vi "Test.vi"() -> ()   [LabVIEW 2018]
uses:
  <vilib>/ethernetip/ethernetip.llb/EthernetIPSLC500FileType.ctl
  <vilib>/ethernetip/ethernetip.llb/EthernetIP SLC500 Read Raw.vi
  <vilib>/ethernetip/ethernetip.llb/EthernetIP SLC500 Write Raw.vi
  <vilib>/ethernetip/ethernetip.llb/EthernetIP SLC500 Write Bit.vi
  <vilib>/ethernetip/ethernetip.lvlib
panel:
  in  "Element Number  2":u16
  in  "Element Number":u16=1
  in  "Bits":bool[](array[boolean])
  in  "Hex Data":u8[](array[numeric]) format="%.0x"
  in  "stop":bool
  out "Input":bool[](array[boolean])
  out "error out":errorcluster
  in  "IP Address":string
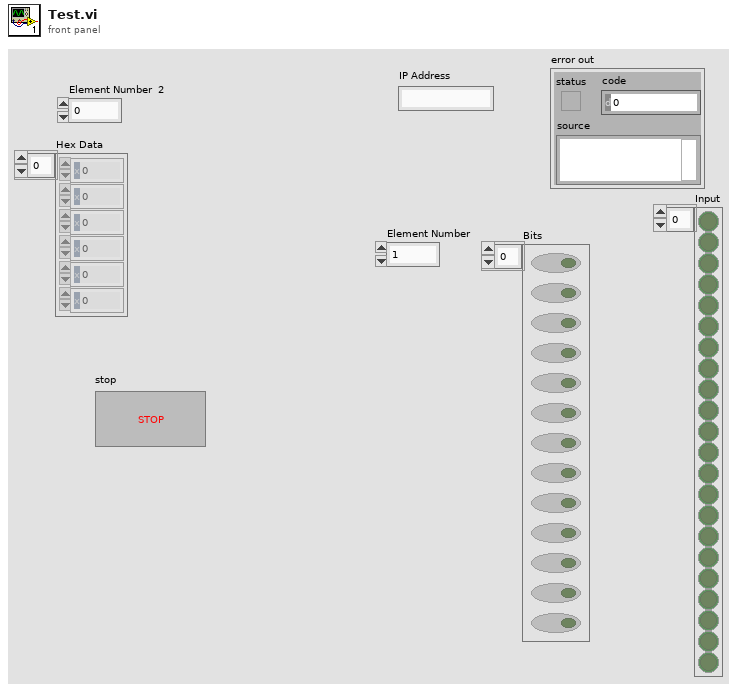
[diagram p1: front panel]
types:
  T1 = typedef "ethernetip.lvlib/ethernetip.ctl" = refnum<k21>
  T2 = typedef "ethernetip.lvlib/EthernetIPSLC500FileType.ctl" = u8
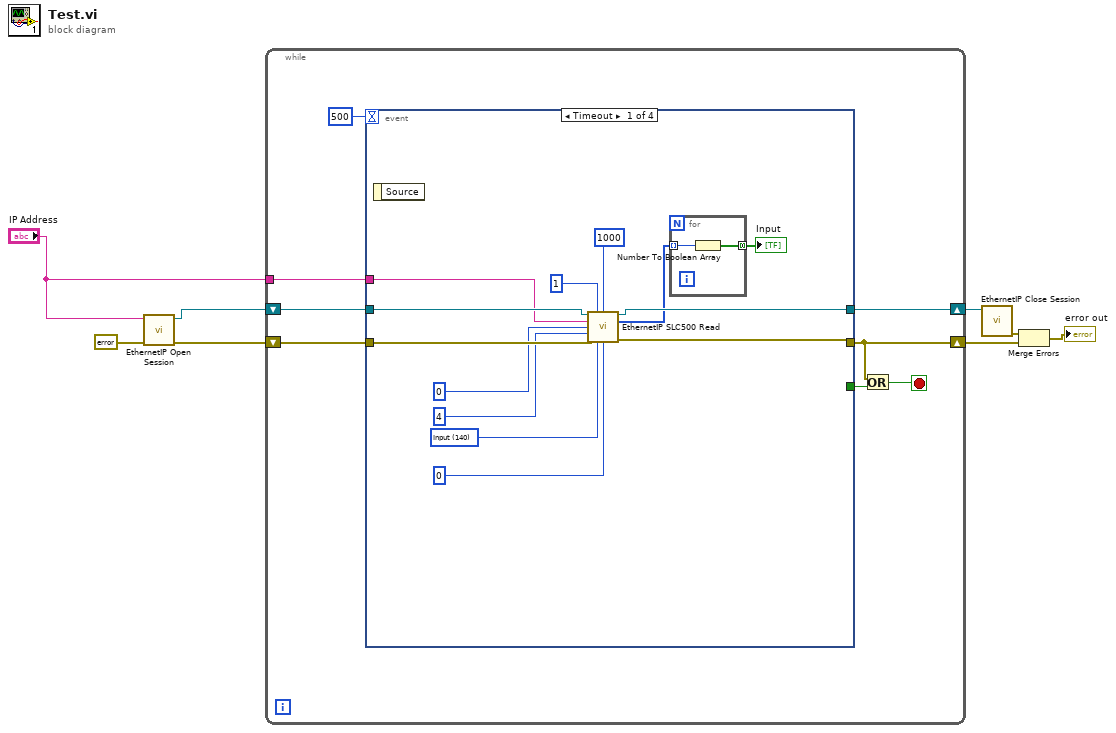
[diagram p0: block diagram]
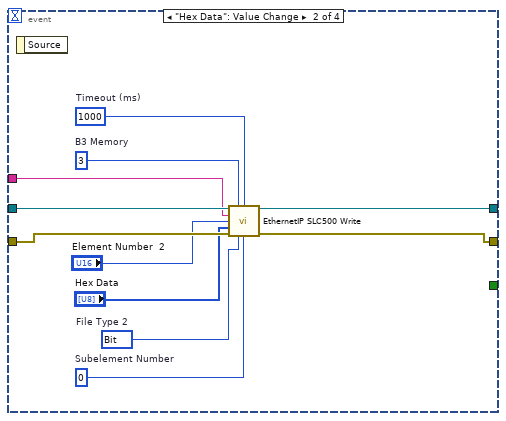
[diagram p2: hidden frame]
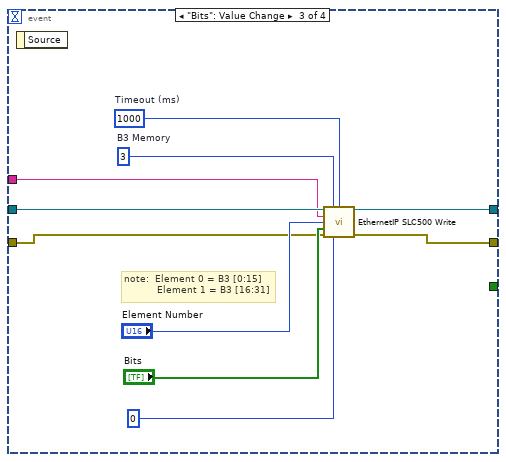
[diagram p3: hidden frame]
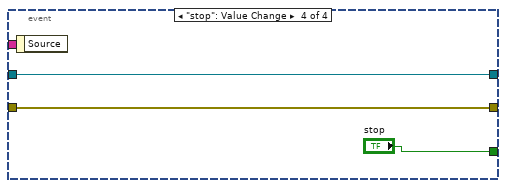
[diagram p4: hidden frame]
diagram:
  n1 = call <vilib>:"EthernetIP Open Session.vi"("error in"=errorcluster {"status"=FALSE, "code"=0, "source"=""} ("error in (no error)"), "Session in"="IP Address") -> ("error out"=w4:errorcluster, "Session out"=w3:T1)  [unwired: 8 in]
  n2 = while {
    shift-right: [w10] -> w6
    shift-left: w4 -> [w13]
    shift-right: [w11] -> w2
    shift-left: w3 -> [w12]
    tunnel: "IP Address" -> [w9]
    stop <- w14 stop-if-true
    n3 = event shown="[0] Timeout" {
      selector: _ -> [_ _ _ _]
      dyn-events: _ -> [_ _ _ _]
      timeout: 500 -> [_ _ _ _]
      tunnel: [_ _ _ "stop"] -> w15
      tunnel: w13 -> [w28 w40 w47 w54]
      tunnel: [w26 w39 w46 w54] -> w10
      tunnel: w12 -> [w29 w42 w50 w53]
      tunnel: [w27 w41 w49 w53] -> w11
      tunnel: w9 -> [w25 w36 w48 _]
      event Timeout {
        w18 = T2 140 items=["Status"=132, "Bit"=133, "Timer"=134, "Counter"=135, "Control"=136, "Integer"=137, "Float"=138, "Output"=139, "Input"=140, "String"=141, "ASCII"=142] ("File Type")
        n4 = event-data() -> ()  [unwired: 1 in, 1 out]
        n5 = call-poly <vilib>:"EthernetIP SLC500 Read.vi"("Session in"=w29, "File Number"=u16 1, "Timeout (ms)"=1000, "Network Path"=w25, "Element Number"=u16 0, "Number of Bytes"=u32 4, "error in"=w28, "File Type"=w18, "Subelement Number"=u16 0) -> ("Session out"=w27:T1, "Data"=w21:u8[], "error out"=w26:errorcluster)  [unwired: 4 in]
        n6 = for {
          tunnel: w21 -> [w31] mode=indexing
          tunnel: [w30] -> w22 mode=concatenating
          n7 = Number To Boolean Array(number=w31) -> (Boolean array=w30:bool[])
        }
        "Input" <- w22
      }
      event "Hex Data": Value Change {
        w32 = u16 0  # Subelement Number
        w33 = T2 133 items=["Status"=132, "Bit"=133, "Timer"=134, "Counter"=135, "Control"=136, "Integer"=137, "Float"=138, "Output"=139, "Input"=140, "String"=141, "ASCII"=142]  # File Type 2
        w37 = u16 3  # B3 Memory
        w38 = 1000  # Timeout (ms)
        n8 = event-data() -> ()  [unwired: 1 in, 1 out]
        n9 = call-poly <vilib>:"EthernetIP SLC500 Write.vi"("Session in"=w42, "File Number"=w37, "Timeout (ms)"=w38, "Network Path"=w36, "Element Number"="Element Number  2", "Data"="Hex Data", "error in"=w40, "File Type"=w33, "Subelement Number"=w32) -> ("Session out"=w41:T1, "error out"=w39:errorcluster)  [unwired: 5 in]
      }
      event "Bits": Value Change {
        w44 = 1000  # Timeout (ms)
        w45 = u16 3  # B3 Memory
        # "note:  Element 0 = B3 [0:15]\n           Element 1 = B3 [16:31]"
        n10 = event-data() -> ()  [unwired: 1 in, 1 out]
        n11 = call-poly <vilib>:"EthernetIP SLC500 Write.vi"("Session in"=w50, "File Number"=w45, "Timeout (ms)"=w44, "Network Path"=w48, "Element Number"="Element Number", "Data"="Bits", "error in"=w47, "Bit Offset"=u16 0) -> ("Session out"=w49:T1, "error out"=w46:errorcluster)  [unwired: 6 in]
      }
      event "stop": Value Change {
        n12 = event-data() -> ()  [unwired: 1 in, 1 out]
      }
    }
    n13 = Or(x=w10, y=w15) -> (x .or. y?=w14:bool)
  }
  n14 = call <vilib>:"EthernetIP Close Session.vi"("Session in"=w2) -> ("error out"=w8:errorcluster)  [unwired: 10 in]
  n15 = Merge Errors(w8, w6) -> (→"error out":errorcluster)
